vi "add_available_methods.vi"() -> ()   [LabVIEW 2020]
uses:
  <vilib>/regexp/Match Regular Expression.xnode
panel:
  out "concatenated string":string
  out "vi path":path
  out "error out 2":errorcluster
  out "Array 4":string[][](array[string])
  out "error out":errorcluster
  out "path":path
  out "text":string
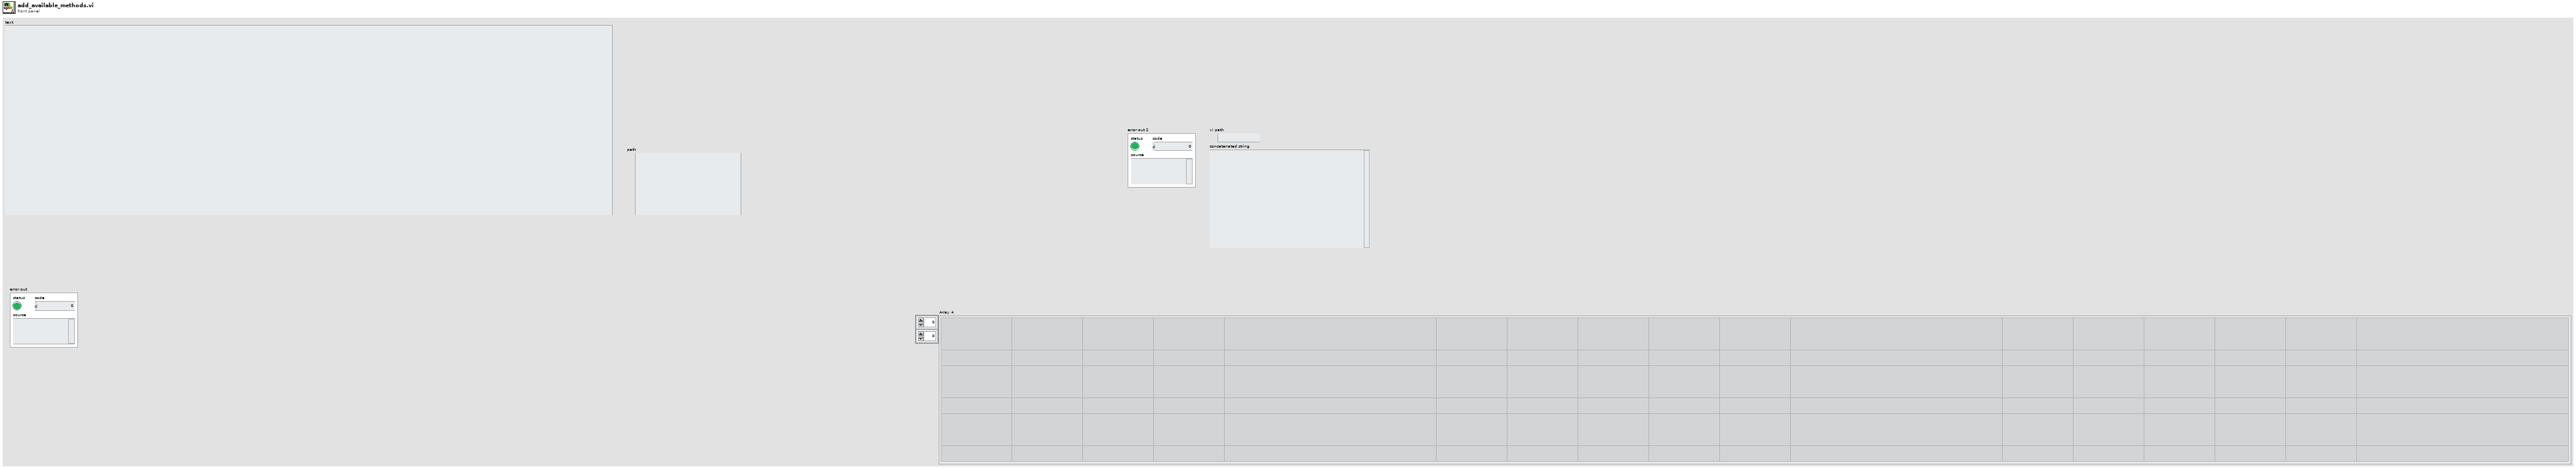
[diagram p1: front panel]
types:
  T1 = enum16{"open", "replace", "create", "open or create", "replace or create", "replace or create with confirmation"}
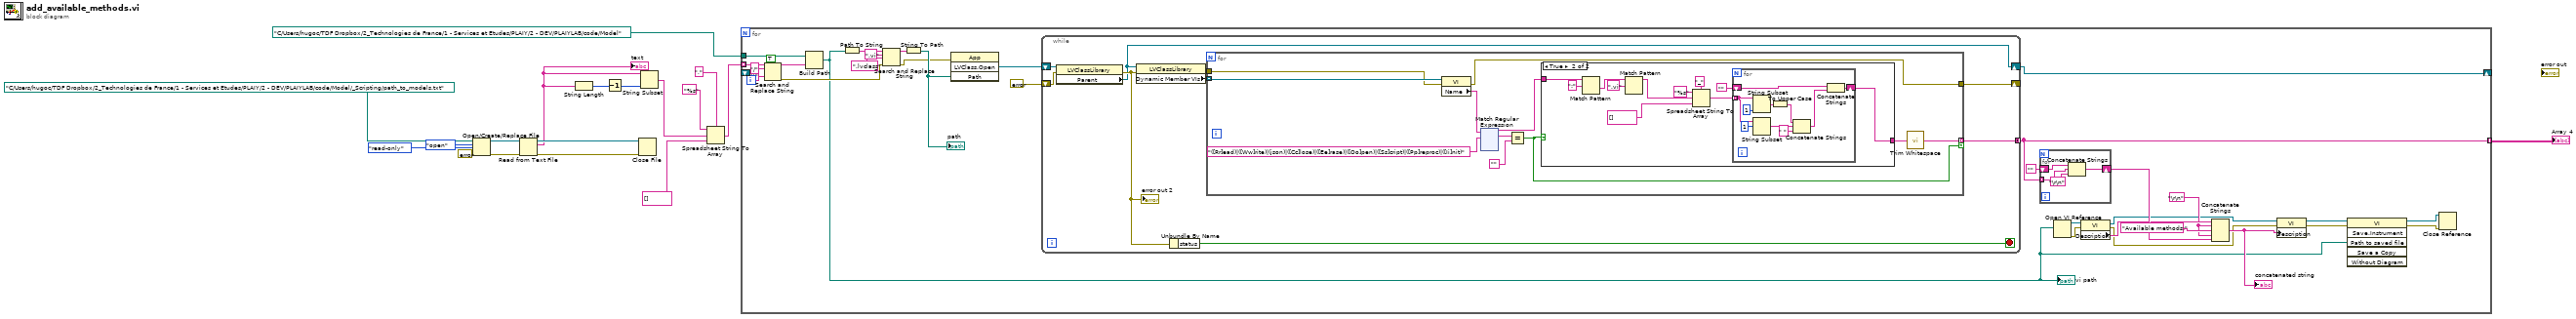
[diagram p0: block diagram]
diagram:
  n1 = Open/Create/Replace File(file path (use dialog)=path "C:/Users/hugoc/TDF Dropbox/2_Technologies de France/1 - Services et Etudes/PLAIY/2 - DEV/PLAIYLAB/code/Model/_Scripting/path_to_models.txt", error in=errorcluster {"status"=FALSE, "code"=0, "source"=""}, operation (0:open)=T1."open", access (0:read/write)=enum16{"read/write", "read-only", "write-only"}."read-only") -> (refnum out=w14:refnum<file>, error out=w13:errorcluster)  [unwired: 2 in, 1 out]
  n2 = Read from Text File(file (use dialog)=w14, error in=w13) -> (refnum out=w12:refnum<file>, text=w4:string, error out=w11:errorcluster)  [unwired: 2 in, 1 out]
  "text" <- w4
  n3 = String Length(string=w4) -> (length=w3:i32)
  n4 = Decrement(x=w3) -> (x-1=w2:i32)
  n5 = Close File(refnum=w12, error in=w11) -> ()  [unwired: 2 out]
  n6 = String Subset(string=w4, length (rest)=w2) -> (substring=w5:string)  [unwired: 1 in]
  n7 = Spreadsheet String To Array(delimiter (Tab)=",", format string="%s", spreadsheet string=w5, array type (2D Dbl)=string[] []) -> (array=w7:string[])
  n8 = for {
    tunnel: w7 -> [w43] mode=indexing
    tunnel: path "C:/Users/hugoc/TDF Dropbox/2_Technologies de France/1 - Services et Etudes/PLAIY/2 - DEV/PLAIYLAB/code/Model" -> [w46]
    shift-right: [w35] -> _
    shift-left: _ -> [_]
    tunnel: [w33] -> w1 mode=indexing
    w28 = "\r\n"
    n9 = Search and Replace String(replace all?=TRUE ("replace all? (F)"), input string=w43, search string="/", replace string="\\" ("replace string (\"\")")) -> (result string=w40:string, error out=w39:errorcluster)  [unwired: 4 in, 2 out]
    n10 = Build Path(base path=w46, name or relative path=w40) -> (appended path=w24:path)
    "vi path" <- w24
    n11 = Path To String(path=w24) -> (string=w48:string)
    n12 = Search and Replace String(input string=w48, search string=".vi", replace string=".lvclass" ("replace string (\"\")"), error in=w39) -> (result string=w47:string, error out=w38:errorcluster)  [unwired: 4 in, 2 out]
    n13 = String To Path(string=w47) -> (path=w45:path)
    "path" <- w45
    n14 = invoke class="App" method="LVClass.Open"(error in=w38, "Path"=w45) -> ("LVClass.Open"=w37:refnum<vi>)  [unwired: 2 in, 3 out]
    n15 = while {
      shift-right: [w57] -> _
      shift-left: errorcluster {"status"=FALSE, "code"=0, "source"=""} ("error in (no error)") -> [w61]
      shift-right: [w56] -> w35
      shift-left: w37 -> [w62]
      tunnel: [w55] -> w33 mode=concatenating
      stop <- w59 stop-if-true
      n16 = property class="LVClassLibrary"(reference=w62, error in=w61) -> (error out=w60:errorcluster, "Parent"=w56:refnum<vi>)  [unwired: 1 out]
      "error out 2" <- w60
      n17 = property class="LVClassLibrary"(reference=w56, error in=w60) -> (error out=w58:errorcluster, "Dynamic Member VIs"=w63:refnum<vi>[])  [unwired: 1 out]
      n18 = Unbundle By Name(w60) -> ("status"=w59:bool)
      n19 = for {
        tunnel: w63 -> [w74] mode=indexing
        tunnel: w58 -> [w73]
        tunnel: [w67] -> w57
        tunnel: [w64] -> w55 mode=indexing if=w66
        n20 = property class="VI"(reference=w74, error in=w73) -> (error out=w67:errorcluster, "Name"=w65:string)  [unwired: 1 out]
        n21 = xnode "Match Regular Expression"("input string"=w65, "regular expression"="([Rr]ead)|([Ww]rite)|(json)|([Cc]lose)|([Ee]rase)|([Oo]pen)|([Ss]cript)|([Pp]reproc)|([Ii]nit)") -> ("before match"=w69:string, "whole match"=w71:string)  [unwired: 4 in, 3 out]
        n22 = Equal?(x=w71, y="") -> (x = y?=w66:bool)
        n23 = case shown="True" w66 {
          tunnel: w69 -> [w189 w200]
          tunnel: [w189 w190] -> w68
          frame False {
          }
          frame True {
            n24 = Match Pattern(string=w200, regular expression=":") -> (after substring=w198:string)  [unwired: 1 in, 3 out]
            n25 = Match Pattern(string=w198, regular expression=".vi") -> (before substring=w196:string)  [unwired: 1 in, 3 out]
            n26 = Spreadsheet String To Array(delimiter (Tab)="_", format string="%s", spreadsheet string=w196, array type (2D Dbl)=string[] []) -> (array=w192:string[])
            n27 = for {
              tunnel: w192 -> [w209] mode=indexing
              shift-right: [w202] -> w190
              shift-left: "" -> [w206]
              n28 = String Subset(string=w209, length (rest)=1 ("length (rest)")) -> (substring=w207:string)  [unwired: 1 in]
              n29 = String Subset(string=w209, offset (0)=1) -> (substring=w204:string)  [unwired: 1 in]
              n30 = To Upper Case(1:w207) -> (0:w205:string)
              n31 = Concatenate Strings(w205, w204, " " ("string")) -> (w203:string)
              n32 = Concatenate Strings(w206, w203) -> (w202:string)
            }
          }
        }
        n33 = call <vilib>:"Trim Whitespace.vi"("string"=w68) -> ("trimmed string"=w64:string)  [unwired: 1 in]
      }
    }
    n34 = for {
      tunnel: w33 -> [w51] mode=indexing
      shift-right: [w53] -> w31
      shift-left: "" -> [w52]
      n35 = Concatenate Strings(w52, w51, "\r\n") -> (w53:string)
    }
    n36 = Open VI Reference(vi path=w24) -> (vi reference=w34:refnum<vi>, error out=w19:errorcluster)  [unwired: 5 in]
    n37 = property class="VI"(reference=w34, error in=w19) -> (reference out=w27:refnum<vi>, error out=w20:errorcluster, "Description"=w30:string)
    n38 = Concatenate Strings(w30, w28, "Available methods:" ("string"), w28, w31) -> (w26:string)
    "concatenated string" <- w26
    n39 = property class="VI"(reference=w27, error in=w20, "Description"=w26) -> (reference out=w25:refnum<vi>, error out=w21:errorcluster)
    n40 = invoke class="VI" method="Save.Instrument"(reference=w25, error in=w21, "Path to saved file"=w24) -> (reference out=w23:refnum<vi>, error out=w22:errorcluster)  [unwired: 3 in, 4 out]
    n41 = Close Reference(reference=w23, error in (no error)=w22) -> ()  [unwired: 1 out]
  }
  "Array 4" <- w1
